vi "degree_to_radian__v1.vi"(11 "degree":ext) -> (3 "radian":ext)   [LabVIEW 2020]
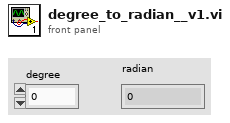
[diagram p1: front panel]
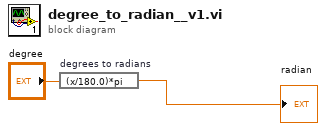
[diagram p0: block diagram]
diagram:
  n1 = expression code="(x/180.0)*pi" "degrees to radians"("degree") -> (→"radian":ext)
